vi "latchTest.vi"() -> ()   [LabVIEW 2014]
panel:
  out "Boolean 2":bool
  in  "Boolean":bool
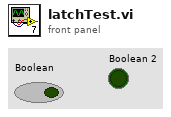
[diagram p1: front panel]
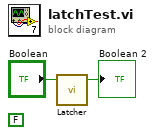
[diagram p0: block diagram]
diagram:
  (unwired) FALSE
  n1 = call "Latcher.vi"("Value In"="Boolean") -> ("Latched"=→"Boolean 2":bool)  [unwired: 4 in]
